vi "FG Set New LocalPose.vi"(1 "FG Action (Read)":T1, 2 "Set New LocalPose In":bool) -> (0 "Set New LocalPose Out":bool)   [LabVIEW 2009]
uses:
  cRIO/Functional Global Variables/Actions for FG's.ctl
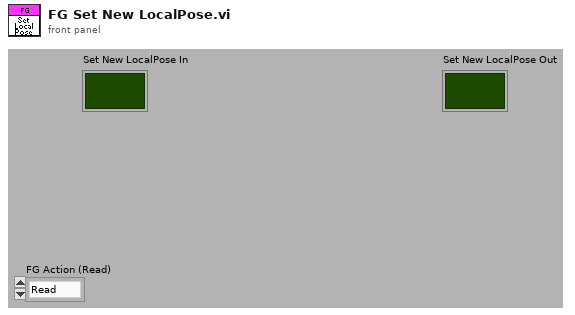
[diagram p1: front panel]
types:
  T1 = typedef "Actions for FG's.ctl" = enum16{"Read", "Write"}
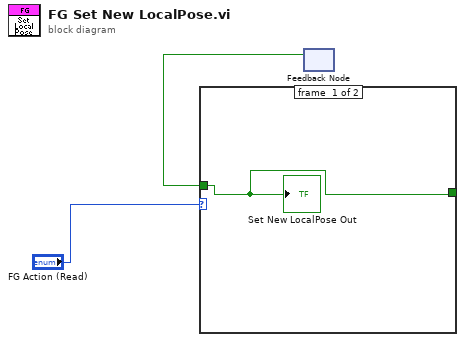
[diagram p0: block diagram]
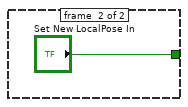
[diagram p2: hidden frame]
diagram:
  n1 = feedback #1() -> (w1:bool)  [unwired: 1 in]
  n2 = case shown="\"Write\"" "FG Action (Read)" {
    tunnel: [w4 "Set New LocalPose In"] -> w2
    tunnel: w1 -> [w4 _]
    frame #0 {
      "Set New LocalPose Out" <- w4
    }
    frame #1 {
    }
  }
